vi "Check Valves.vi"(8 "error in (no error)":errorcluster, 11 "ValveControlModule in":refnum<class "DigitalControlModule.lvclass">) -> (0 "error out":errorcluster, 3 "ValveControlModule out":refnum<class "DigitalControlModule.lvclass">)   [LabVIEW 2020, in "VolatusControl.lvlib" / "DigitalControlModule.lvclass"]
uses:
  DigitalControlModule.lvclass
  DigitalControlModule.lvclass/DigitalControlModule.ctl
  Volatus/MessageQ/MessageQ.lvclass
  Valve Action.ctl
  VolatusControl.lvlib
  <vilib>/Utility/miscctls.llb/LVMapReplaceAction.ctl
  messages/CmdDigital/Data.ctl
  messages/CmdDigital/CmdDigital.lvlib
  messages/CmdDigitalMultiple/Data.ctl
  messages/CmdDigitalMultiple/CmdDigitalMultiple.lvlib
  DigitalControl/DigitalControl.lvclass
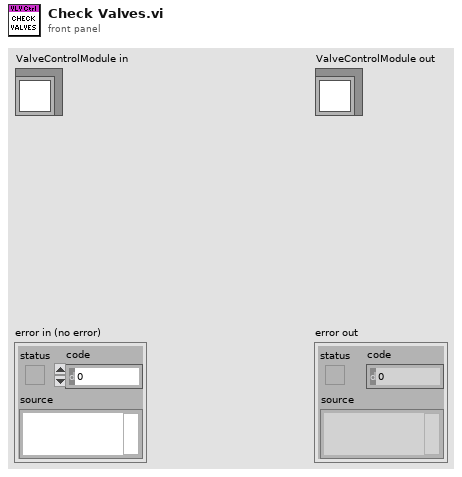
[diagram p1: front panel]
types:
  T1 = typedef "VolatusControl.lvlib/Valve Action.ctl" = cluster{"Channel":string, "MsgQ":refnum<class "MessageQ.lvclass">, "Value":bool}
  T2 = typedef "LVMapReplaceAction.ctl" = enum32{"Modify Entry only if found", "Add or Modify Entry", "Delete Entry"}
  T3 = map{string, refnum<class "DigitalControl.lvclass">}
  T4 = typedef "CmdDigitalMultiple.lvlib/Data.ctl" = cluster{"values":T5[]}
  T5 = typedef "CmdDigital.lvlib/Data.ctl" = cluster{"channel":string, "value":bool}
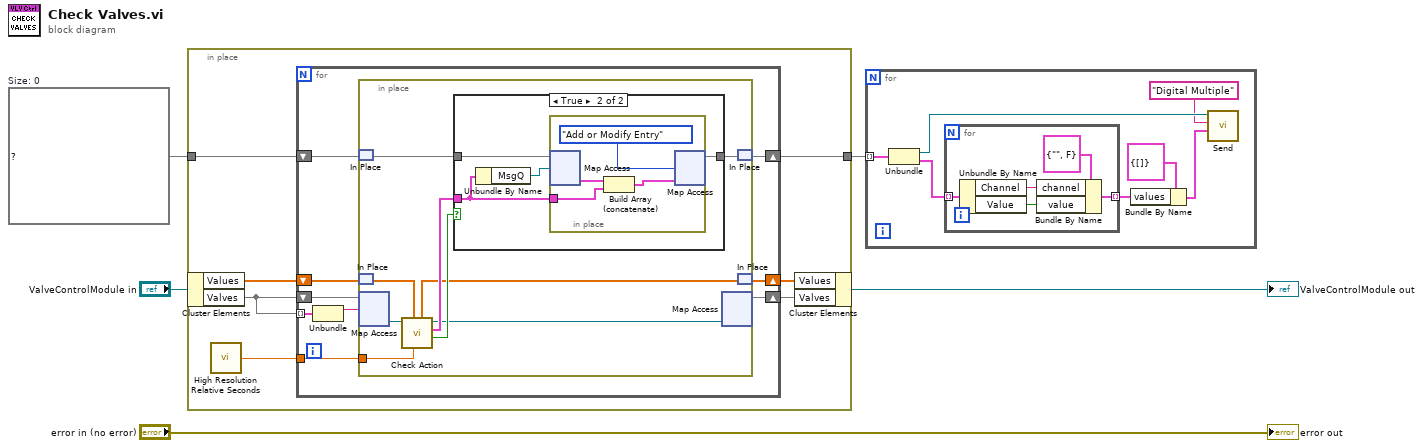
[diagram p0: block diagram]
diagram:
  w3 = map{refnum<class "MessageQ.lvclass">, T1[]} {}  # Size: 0
  n1 = in-place {
    in-place-border: w3 -> [w10]
    in-place-border: [w8] -> w1
    n2 = in-place-cluster #1("ValveControlModule in") -> ("Values"=w7:dbl[], "Valves"=w12:T3)
    n3 = call <vilib>:"High Resolution Relative Seconds.vi"() -> ("relative seconds"=w11:dbl)
    n4 = for {
      shift-right: [w17] -> w9
      shift-left: w12 -> [w20]
      tunnel: w12 -> [w21] mode=indexing
      tunnel: w11 -> [w18]
      shift-right: [w14] -> w8
      shift-left: w10 -> [w15]
      shift-right: [w13] -> w6
      shift-left: w7 -> [w16]
      n5 = Unbundle(w21) -> ("Name"=w19:string)  [unwired: 1 out]
      n6 = in-place {
        in-place-border: w18 -> [w29]
        n7 = in-place-match #2(w15) -> (w25:map{refnum<class "MessageQ.lvclass">, T1[]})
        n8 = in-place-match #3(w16) -> (w23:dbl[])
        n9 = in-place-map #4(w20, w19) -> (w30:refnum<class "DigitalControl.lvclass">)  [unwired: 1 in, 1 out]
        n10 = call-dynamic "Check Action.vi"("HRS Time"=w29, "Values In"=w23, "Valve in"=w30) -> ("Do Action"=w28:bool, "Action"=w27:T1, "Valve out"=w26:refnum<class "DigitalControl.lvclass">, "Values"=w22:dbl[])  [unwired: 4 in, 1 out]
        n11 = case shown="True" w28 {
          tunnel: w27 -> [_ w33]
          tunnel: w25 -> [w31 w35]
          tunnel: [w31 w32] -> w24
          frame False {
          }
          frame True {
            n12 = Unbundle By Name(w33) -> ("MsgQ"=w34:refnum<class "MessageQ.lvclass">)
            n13 = in-place {
              in-place-border: w33 -> [w38]
              n14 = in-place-map #5(w35, w34) -> (w39:T1[])  [unwired: 1 in, 1 out]
              n15 = Build Array (concatenate)(w39, w38) -> (w37:T1[])
              n16 = in-place-map #5(w37, LVMapReplaceAction."Add or Modify Entry" ("action")) -> (w32:map{refnum<class "MessageQ.lvclass">, T1[]})  [unwired: 2 out]
            }
          }
        }
        n17 = in-place-map #4(w26) -> (w17:T3)  [unwired: 1 in, 2 out]
        n18 = in-place-match #2(w24) -> (w14:map{refnum<class "MessageQ.lvclass">, T1[]})
        n19 = in-place-match #3(w22) -> (w13:dbl[])
      }
    }
    n20 = in-place-cluster #1("Values"=w6, "Valves"=w9) -> (→"ValveControlModule out":refnum<class "DigitalControlModule.lvclass">)
  }
  n21 = for {
    tunnel: w1 -> [w46] mode=indexing
    n22 = Unbundle(w46) -> ("Volatus:MessageQ"=w42:refnum<class "MessageQ.lvclass">, "Array"=w45:T1[])
    n23 = for {
      tunnel: w45 -> [w51] mode=indexing
      tunnel: [w47] -> w43 mode=indexing
      n24 = Unbundle By Name(w51) -> ("Channel"=w49:string, "Value"=w48:bool)
      n25 = Bundle By Name(cluster=T5 {"channel"="", "value"=FALSE} ("CmdDigital"), "channel"=w49, "value"=w48) -> (w47:T5)
    }
    n26 = Bundle By Name(cluster=T4 {"values"=[]} ("CmdDigitalMultiple"), "values"=w43) -> (w41:T4)
    n27 = call "Send.vi"("Data"=w41, "ID"="Digital Multiple", "MessageQ in"=w42) -> ()  [unwired: 7 in, 2 out]
  }
  "error out" <- "error in (no error)"
